vi "Photovoltaic.vi"() -> ()   [LabVIEW 2018]
uses:
  <vilib>/OPCUA/controls/NodeIds.ctl
  <vilib>/OPCUA/controls/NodeId.ctl
  GlobalVal.vi
  <vilib>/OPCUA/client/Multiple Read Variant.vi
  <vilib>/OPCUA/NI OPC UA Client.lvlib
panel:
  in  "PV001_Ki":dbl
  in  "PV001_Kp":dbl
  in  "PV001_tp":dbl
  in  "PV001_kP":dbl
  in  "PV001_tf":dbl
  in  "PV001_kf":dbl
  out "PT001_tf":dbl
  out "DS001_Ki":dbl
  out "PT001_tP":dbl caption="DS001_tP"
  out "PT001_kf":dbl caption="DS001_kf"
  out "PT001_kP":dbl caption="DS001_kP"
  out "BT001_Kp":dbl caption="DS001_Kp"
  out "PV001_Thermo":dbl(slide) scale=0.0..100.0
  out "Photovoltaic":dbl(knob) scale=0.0..100.0
  out "OPCUA Error Log":errorcluster
  out "OPC Server URL":string
  out "PV001_f0, f Chart":cluster{dbl, dbl}(graph)
  out "PV001_P0, P Chart":cluster{dbl, dbl}(graph)
  out "Time Stamp":timestamp
  out "Pmin":dbl(slide) scale=10.0..60.0
  out "Pmax":dbl(slide) scale=10.0..60.0
  in  "stop":bool
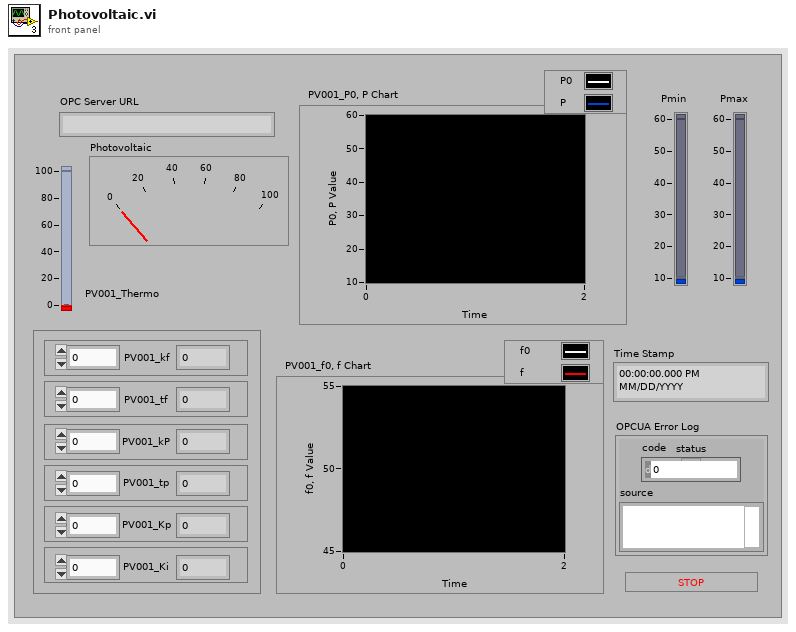
[diagram p1: front panel]
types:
  T1 = typedef "OPC UA Client Refnum.ctl" = refnum<k21>
  T2 = typedef "NodeIds.ctl" = T3[]
  T3 = typedef "NodeId.ctl" = string
  T4 = typedef "Read Variant Result.ctl" = cluster{"node ID":T3, "value ":variant, "timestamp":timestamp, "status":T5}
  T5 = typedef "OPC UA StatusCode.ctl" = u32
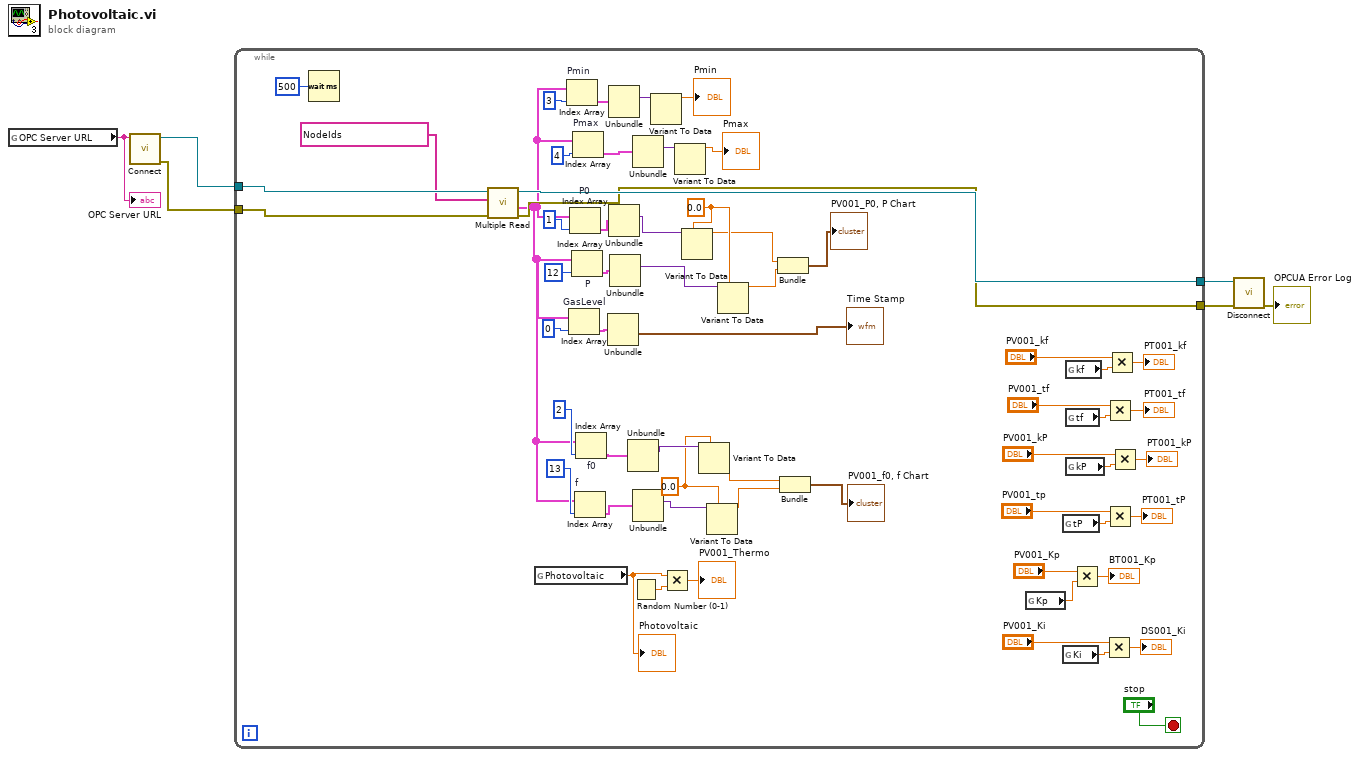
[diagram p0: block diagram]
diagram:
  n1 = global read "GlobalVal.vi" "OPC Server URL"() -> (w1:string)
  "OPC Server URL" <- w1
  n2 = call <vilib>:"Connect.vi"("server endpoint URL"=w1) -> ("error out"=w5:errorcluster, "OPC UA client refnum out"=w6:T1)  [unwired: 8 in, 1 out]
  n3 = while {
    tunnel: w6 -> [w65]
    tunnel: w5 -> [w64]
    tunnel: [w62] -> w4
    tunnel: [w61] -> w3
    stop <- "stop" stop-if-true
    w32 = 0.0
    w42 = 0.0
    n4 = Wait (ms)(milliseconds to wait=u32 500) -> ()  [unwired: 1 out]
    n5 = call-poly <vilib>:"Multiple Read.vi"("error in (no error)"=w64, "node IDs"=T2 ["ns=2;i=2", "ns=2;i=3", "ns=2;i=4", "ns=2;i=5", "ns=2;i=6", "ns=2;i=7", "ns=2;i=8", "ns=2;i=9", "ns=2;i=10", "ns=2;i=11", "ns=2;i=12", "ns=2;i=13", "ns=2;i=14", "ns=2;i=15"], "OPC UA client refnum in"=w65) -> ("error out"=w61:errorcluster, "results"=w28:T4[], "OPC UA client refnum out"=w62:T1)  [unwired: 5 in, 1 out]
    n6 = global read "GlobalVal.vi" "Photovoltaic"() -> (w27:dbl)
    "Photovoltaic" <- w27
    n7 = Index Array "Pmin"(array=w28, index=3) -> (element=w54:T4)
    n8 = Index Array "GasLevel"(array=w28, index=0) -> (element=w58:T4)
    n9 = Index Array "P0"(array=w28, index=1) -> (element=w56:T4)
    n10 = Index Array "P"(array=w28, index=12) -> (element=w45:T4)
    n11 = Index Array "Pmax"(array=w28, index=4) -> (element=w50:T4)
    n12 = Index Array "f"(array=w28, index=13) -> (element=w34:T4)
    n13 = Index Array "f0"(array=w28, index=2) -> (element=w37:T4)
    n14 = Unbundle(w58) -> ("timestamp"=→"Time Stamp":timestamp)  [unwired: 3 out]
    n15 = Unbundle(w54) -> ("value"=w53:variant)  [unwired: 3 out]
    n16 = Unbundle(w56) -> ("value"=w44:variant)  [unwired: 3 out]
    n17 = Unbundle(w45) -> ("value"=w43:variant)  [unwired: 3 out]
    n18 = Unbundle(w37) -> ("value"=w36:variant)  [unwired: 3 out]
    n19 = Random Number (0-1)() -> (number: 0 to 1=w26:dbl)
    n20 = Unbundle(w50) -> ("value"=w49:variant)  [unwired: 3 out]
    n21 = Unbundle(w34) -> ("value"=w33:variant)  [unwired: 3 out]
    n22 = Variant To Data(Variant=w53) -> (data=→"Pmin":dbl)  [unwired: 2 in, 1 out]
    n23 = Multiply(x=w27, y=w26) -> (x*y=→"PV001_Thermo":dbl)
    n24 = Variant To Data(Variant=w49) -> (data=→"Pmax":dbl)  [unwired: 2 in, 1 out]
    n25 = Variant To Data(type=w42, Variant=w44) -> (data=w39:dbl)  [unwired: 1 in, 1 out]
    n26 = Variant To Data(type=w32, Variant=w36) -> (data=w31:dbl)  [unwired: 1 in, 1 out]
    n27 = Variant To Data(type=w32, Variant=w33) -> (data=w30:dbl)  [unwired: 1 in, 1 out]
    n28 = Variant To Data(type=w42, Variant=w43) -> (data=w40:dbl)  [unwired: 1 in, 1 out]
    n29 = Bundle(w39, w40) -> (→"PV001_P0, P Chart":cluster{dbl, dbl})  [unwired: 1 in]
    n30 = Bundle(w31, w30) -> (→"PV001_f0, f Chart":cluster{dbl, dbl})  [unwired: 1 in]
    n31 = global read "GlobalVal.vi" "Kp"() -> (w11:dbl)
    n32 = global read "GlobalVal.vi" "tP"() -> (w14:dbl)
    n33 = global read "GlobalVal.vi" "Ki"() -> (w7:dbl)
    n34 = global read "GlobalVal.vi" "kf"() -> (w23:dbl)
    n35 = global read "GlobalVal.vi" "tf"() -> (w19:dbl)
    n36 = global read "GlobalVal.vi" "kP"() -> (w16:dbl)
    n37 = Multiply(x="PV001_Kp", y=w11) -> (x*y=→"BT001_Kp":dbl)
    n38 = Multiply(x="PV001_Ki", y=w7) -> (x*y=→"DS001_Ki":dbl)
    n39 = Multiply(x="PV001_tf", y=w19) -> (x*y=→"PT001_tf":dbl)
    n40 = Multiply(x="PV001_tp", y=w14) -> (x*y=→"PT001_tP":dbl)
    n41 = Multiply(x="PV001_kf", y=w23) -> (x*y=→"PT001_kf":dbl)
    n42 = Multiply(x="PV001_kP", y=w16) -> (x*y=→"PT001_kP":dbl)
  }
  n43 = call <vilib>:"Disconnect.vi"("error in (no error)"=w3, "OPC UA client refnum in"=w4) -> ("error out"=→"OPCUA Error Log":errorcluster)  [unwired: 9 in]
